vi "Update Cell Values.vi"(8 "error in (no error)":errorcluster, 10 "Changed Items":T1(array[cluster]), 11 "TreeControl in":refnum<vi>) -> (0 "error out":errorcluster)   [LabVIEW 2013, in "LVTM.lvlib"]
uses:
  LVTM.lvlib
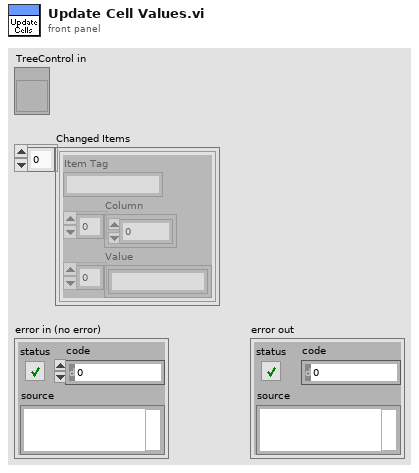
[diagram p1: front panel]
types:
  T1 = cluster{"Item Tag":string, "Column":i32[], "Value":string[]}[]
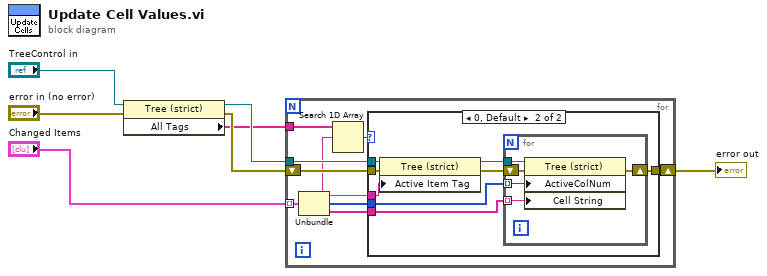
[diagram p0: block diagram]
diagram:
  n1 = property class="Tree (strict)"(reference="TreeControl in", error in="error in (no error)") -> (reference out=w7:refnum<vi>, error out=w4:errorcluster, "All Tags"=w3:string[])
  n2 = for {
    tunnel: "Changed Items" -> [w15] mode=indexing
    shift-right: [w12] -> w1
    shift-left: w4 -> [w16]
    tunnel: w7 -> [w11]
    tunnel: w3 -> [w10]
    n3 = Unbundle(w15) -> ("Item Tag"=w9:string, "Column"=w13:i32[], "Value"=w14:string[])
    n4 = Search 1D Array(1D array=w10, element=w9) -> (index of element=w8:i32)  [unwired: 1 in]
    n5 = case shown="0, Default" w8 {
      tunnel: w16 -> [w17 w23]
      tunnel: w14 -> [_ w22]
      tunnel: w13 -> [_ w21]
      tunnel: [w17 w20] -> w12
      tunnel: w11 -> [_ w19]
      tunnel: w9 -> [_ w18]
      frame -1 {
      }
      frame 0, Default {
        n6 = property on="Property Node" class="Tree (strict)"(reference=w19, error in=w23, "Active Item Tag"=w18) -> (reference out=w24:refnum<vi>, error out=w25:errorcluster)
        n7 = for {
          tunnel: w22 -> [w26] mode=indexing
          tunnel: w21 -> [w27] mode=indexing
          tunnel: w24 -> [w28]
          shift-right: [w29] -> w20
          shift-left: w25 -> [w30]
          n8 = property on="Property Node" class="Tree (strict)"(reference=w28, error in=w30, "ActiveColNum"=w27, "Cell String"=w26) -> (error out=w29:errorcluster)  [unwired: 1 out]
        }
      }
    }
  }
  "error out" <- w1
